vi "Write States.vi"(8 "error in (no error)":errorcluster, 10 "States":T1=enum."PlaceBall", 11 "PlaceBallTactic in":refnum<class "PlaceBallTactic.lvclass">) -> (0 "error out":errorcluster, 3 "PlaceBallTactic out":refnum<class "PlaceBallTactic.lvclass">)   [LabVIEW 2021, in "PlaceBallTactic.lvclass"]
uses:
  PlaceBallTactic.lvclass
  StatesPlaceBallTactic.ctl
  PlaceBallTactic.lvclass/PlaceBallTactic.ctl
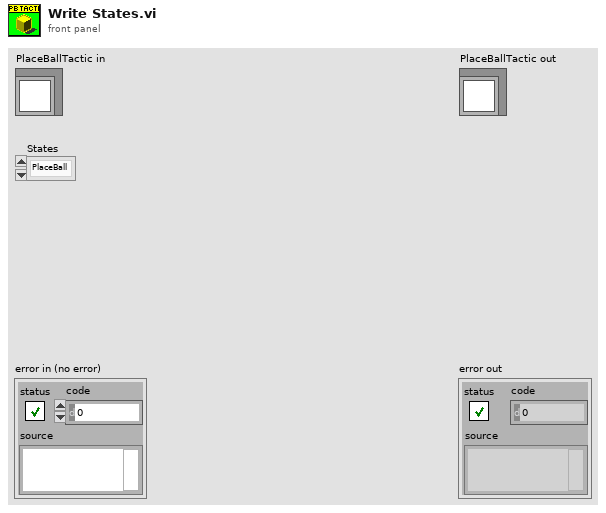
[diagram p1: front panel]
types:
  T1 = typedef "StatesPlaceBallTactic.ctl" = enum16{"GoToGetBall", "PlaceBall", "Exit"}
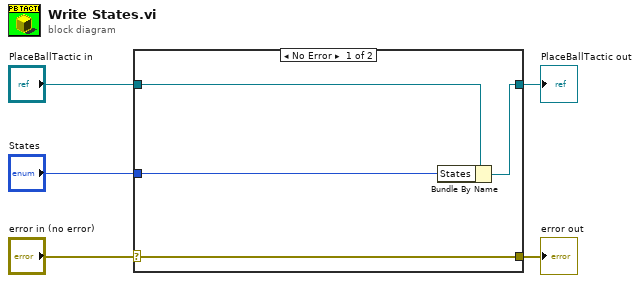
[diagram p0: block diagram]
diagram:
  n1 = case shown="No Error" "error in (no error)" {
    selector: "error in (no error)" -> [w9 w10]
    tunnel: [w9 w10] -> w4
    tunnel: [w7 w11] -> w2
    tunnel: "PlaceBallTactic in" -> [w8 w11]
    tunnel: "States" -> [w6 _]
    frame No Error {
      n2 = Bundle By Name(cluster=w8, "States"=w6) -> (w7:refnum<class "PlaceBallTactic.lvclass">)
    }
    frame Error {
    }
  }
  "error out" <- w4
  "PlaceBallTactic out" <- w2
